vi "TemperatureControl.vi"(8 "error in (no error)":errorcluster, 11 "VISA resource name":refnum<visa-resource-name>="iTC") -> (0 "error out":errorcluster)   [LabVIEW 2021]
uses:
  controls/iTCsetCtrl.ctl
  controls/iTCreadCtrl.ctl
  <vilib>/Instr/_visa.llb/VISA Open Access Mode.ctl
  <vilib>/Utility/file.llb/Write Delimited Spreadsheet (string).vi
panel:
  in  "FilePath":path
  in  "Every (s)":dbl=60.0
  in  "Save Log":bool
  out "Waveform Chart":T1(graph)
  out "Signals":string[](array[string])=["PT1 (K)", "PT2 (K)", "Sample_T (K)", "VTI_T (K)", "Needle Valve (%)", "VTI Heater P", "Sample Heater P ", "VTI Pressure (mBar)"]
  out "Temperature Readings":dbl[](array[numeric])
  in  "Setpoint":dbl
  in  "iTCreadCtrl":T2
  in  "iTCSetCtrl":T3
  in  "Set":bool
  in  "Refresh Time (ms)":i32=100
  in  "Quit":bool
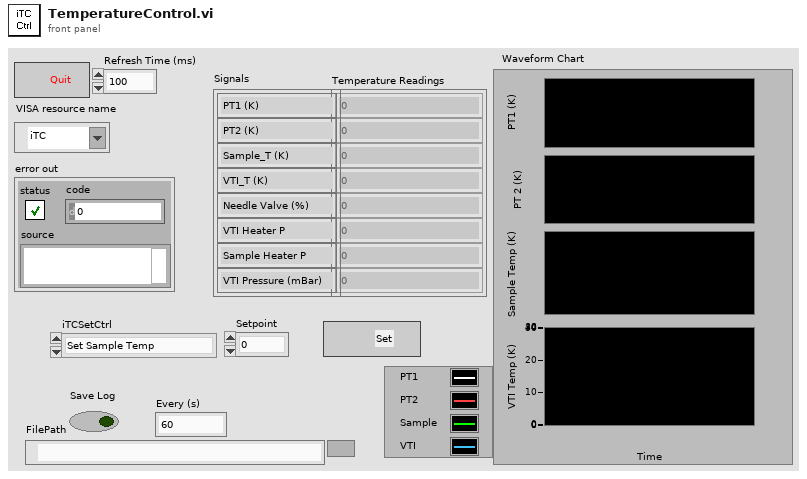
[diagram p1: front panel]
types:
  T1 = cluster{"number":dbl, "number":dbl, "number":dbl, "number":dbl}
  T2 = typedef "iTCreadCtrl.ctl" = enum16{"PT1 Temp", "PT2 Temp", "Sample Temp", "VTI Temp", "Needle Valve", "VTI Heater Power", "Sample Heater Power", "VTI Pressure"}
  T3 = typedef "iTCsetCtrl.ctl" = enum16{"Set Sample Temp", "Set VTI Temp", "Set Needle Valve", "Set VTI Heater Power", "Set Sample Heater Power", "Set VTI Pressure"}
  T4 = typedef "VISA Open Access Mode.ctl" = u32
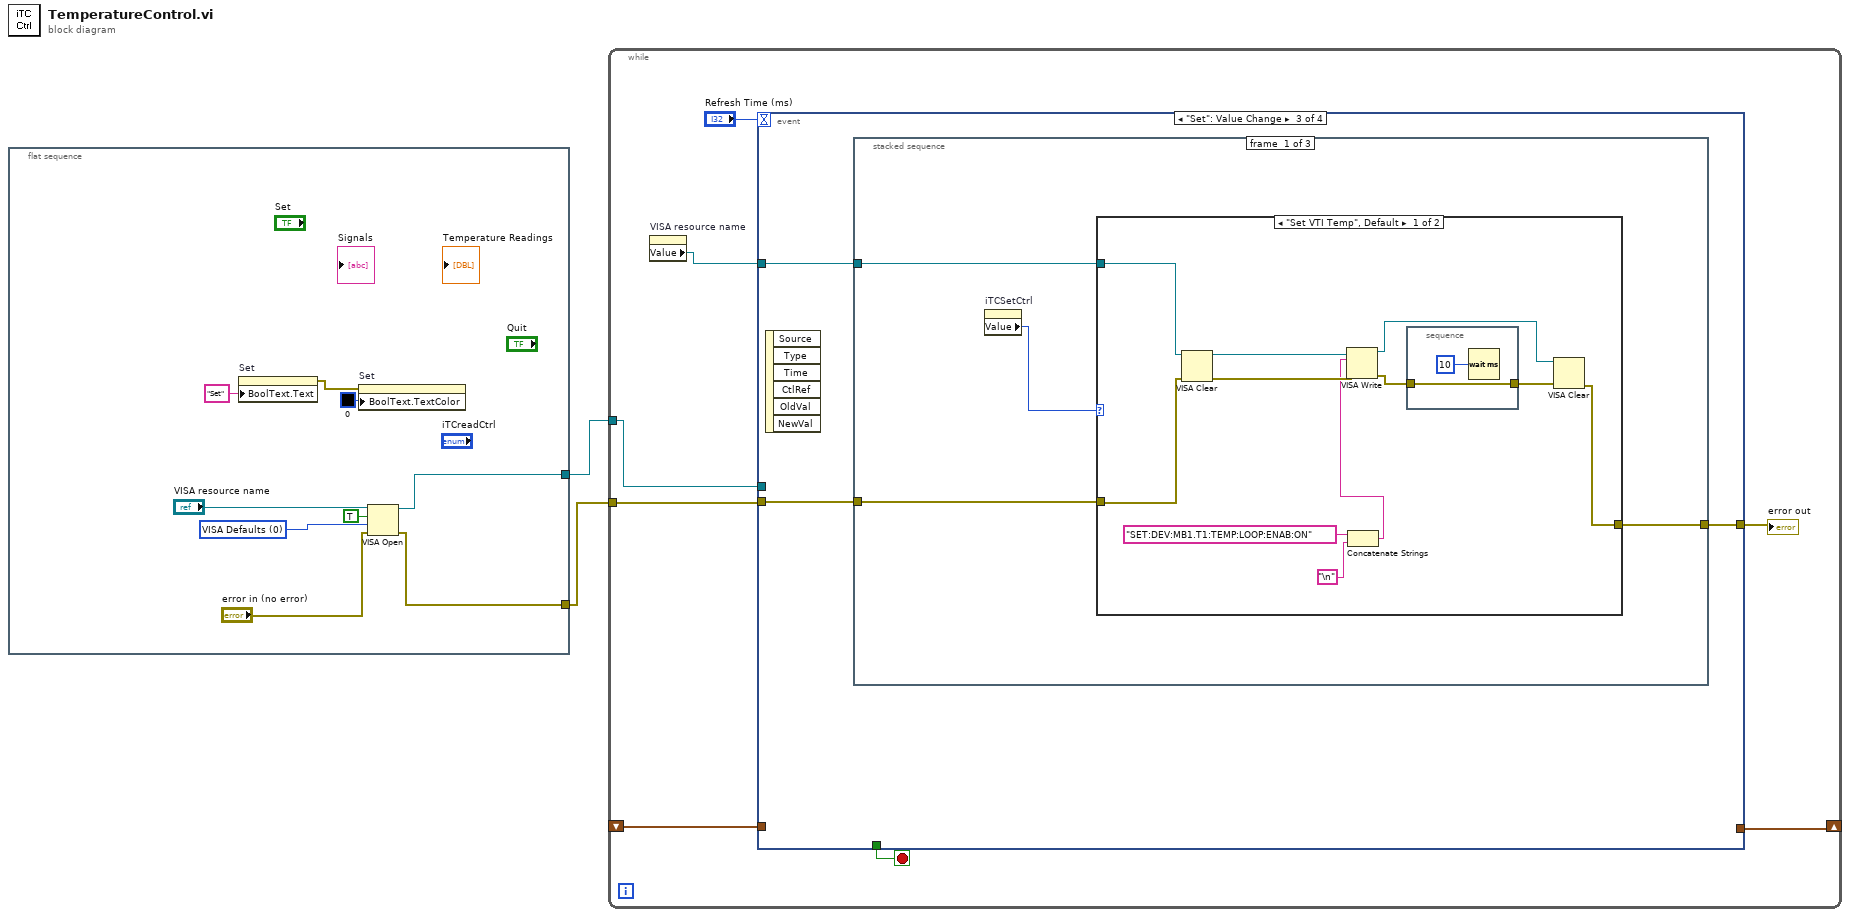
[diagram p0: block diagram]
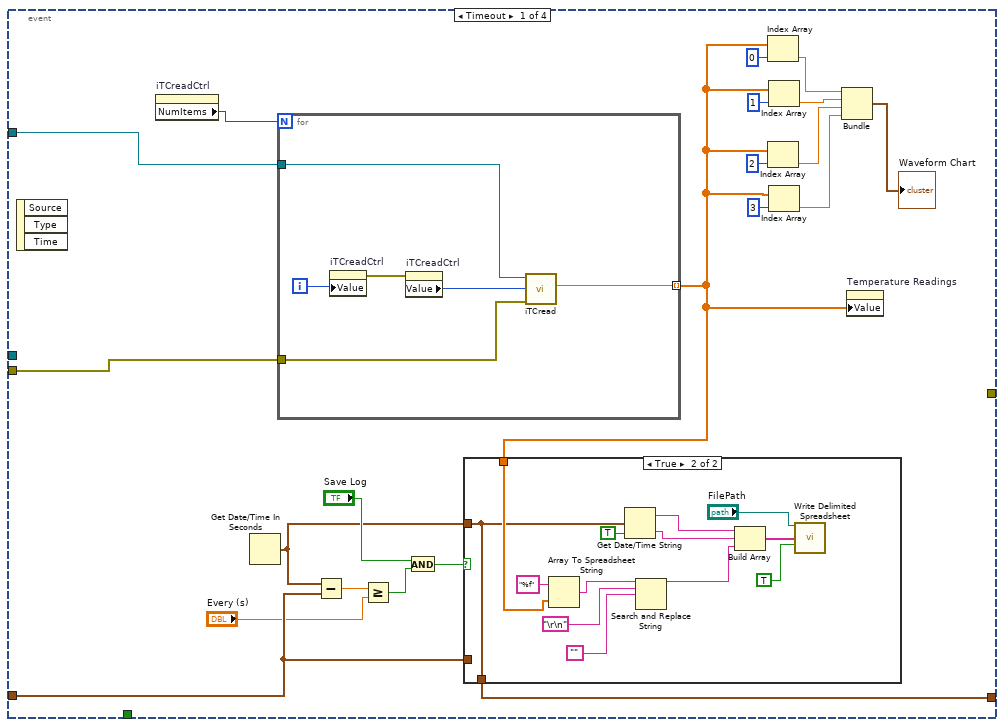
[diagram p2: hidden frame]
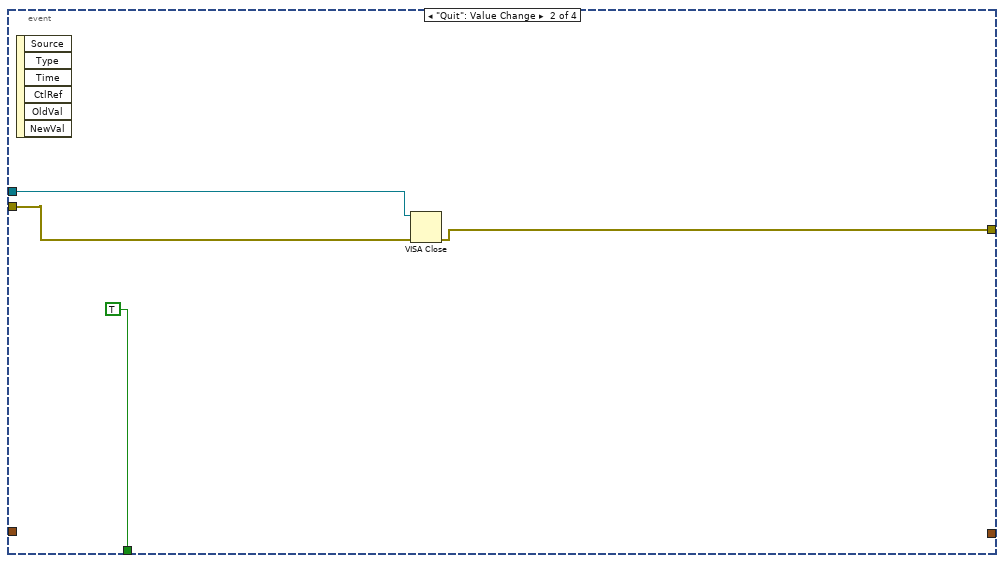
[diagram p4: hidden frame]
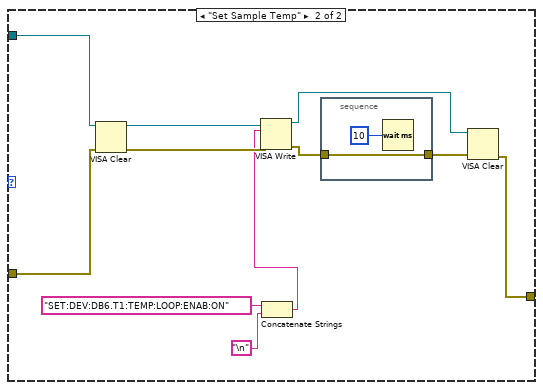
[diagram p5: hidden frame]
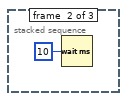
[diagram p6: hidden frame]
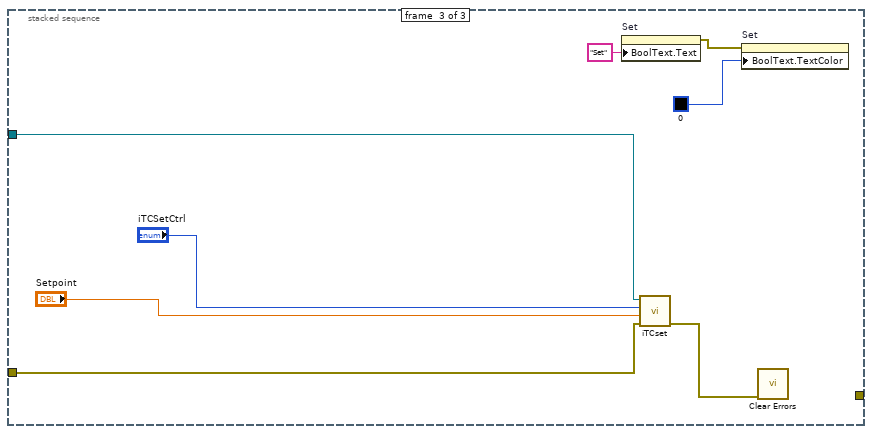
[diagram p7: hidden frame]
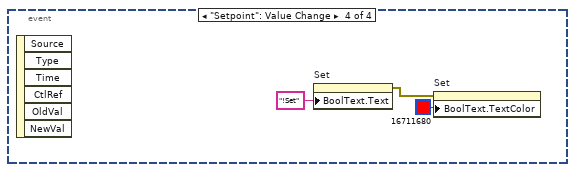
[diagram p8: hidden frame]
diagram:
  n1 = flat-sequence {
    tunnel: [w7] -> w2
    tunnel: [w4] -> w1
    frame #0 {
      w3 = T4 0 items=["VISA Defaults"=0, "Exclusive Lock"=1, "Load Configured Settings"=4] ("Access Mode")
      n2 = property on="Set" class="Bool (strict)"("BoolText.Text"="Set" ("Boolean Text.Text")) -> (error out=w11:errorcluster)  [unwired: 2 in, 1 out]
      n3 = property on="Set" class="Bool (strict)"(error in=w11, "BoolText.TextColor"=u32 0 ("Boolean Text.Colors:BG Color")) -> ()  [unwired: 1 in, 2 out]
      n4 = VISA Open(duplicate session (F)=TRUE, access mode=w3, error in (no error)="error in (no error)", VISA resource name="VISA resource name") -> (VISA resource name=w4:refnum<visa-resource-name>, error out=w7:errorcluster)  [unwired: 1 in]
    }
  }
  n5 = while {
    tunnel: w2 -> [w18]
    tunnel: w1 -> [w15]
    shift-right: [w13] -> _
    shift-left: _ -> [w12]
    stop <- w17 stop-if-true
    n6 = property on="VISA resource name" class="VISAName"() -> ("Value"=w14:refnum<visa-resource-name>)  [unwired: 2 in, 2 out]
    n7 = event shown="[2] \"Set\": Value Change" {
      selector: _ -> [_ _ _ _]
      dyn-events: _ -> [_ _ _ _]
      timeout: "Refresh Time (ms)" -> [_ _ _ _]
      tunnel: w18 -> [w40 w63 w65 _]
      tunnel: [_ w62 w67 _] -> w16
      tunnel: w14 -> [w39 _ w66 _]
      tunnel: [_ TRUE _ _] -> w17
      tunnel: w15 -> [_ w61 _ _]
      tunnel: [w26 _ _ _] -> w13
      tunnel: w12 -> [w25 _ _ _]
      event Timeout {
        n8 = event-data() -> ()  [unwired: 1 in, 3 out]
        n9 = property on="iTCreadCtrl" class="Enum (strict)"() -> ("NumItems"=w38:u32)  [unwired: 2 in, 2 out]
        n10 = Get Date/Time In Seconds() -> (seconds since 1Jan1904=w27:timestamp)
        n11 = for {
          N: w38 -> [_]
          tunnel: w40 -> [w60]
          tunnel: w39 -> [w59]
          tunnel: [w55] -> w20 mode=indexing
          i -> [w58]
          n12 = property on="iTCreadCtrl" class="Enum (strict)"("Value"=w58) -> (error out=w57:errorcluster)  [unwired: 2 in, 1 out]
          n13 = property on="iTCreadCtrl" class="Enum (strict)"(error in=w57) -> ("Value"=w56:T2)  [unwired: 1 in, 2 out]
          n14 = call "iTCread.vi"("VISA resource name"=w59, "iTCreadCtrl"=w56, "error in (no error)"=w60) -> ("number"=w55:dbl)  [unwired: 4 in, 3 out]
        }
        n15 = Subtract(x=w27, y=w25) -> (x-y=w24:dbl)
        n16 = Greater Or Equal?(x=w24, y="Every (s)") -> (x >= y?=w22:bool)
        n17 = And(x="Save Log", y=w22) -> (x .and. y?=w21:bool)
        n18 = case shown="True" w21 {
          tunnel: w27 -> [_ w49]
          tunnel: [w41 w49] -> w26
          tunnel: w25 -> [w41 _]
          tunnel: w20 -> [_ w54]
          frame False {
          }
          frame True {
            n19 = Array To Spreadsheet String(array=w54, 3:"%f" ("format string")) -> (spreadsheet string=w52:string)  [unwired: 1 in]
            n20 = Get Date/Time String(seconds (now)=w49, want seconds? (F)=TRUE ("UTC format")) -> (date string=w47:string, time string=w46:string)  [unwired: 1 in]
            n21 = Search and Replace String(input string=w52, search string="\r\n", replace string="" ("replace string (\"\")")) -> (result string=w45:string)  [unwired: 5 in, 3 out]
            n22 = Build Array(w47, w46, w45) -> (w43:string[])
            n23 = call-poly <vilib>:"Write Delimited Spreadsheet.vi"("file path (dialog if empty)"="FilePath", "1D data"=w43, "append to file? (new file:F)"=TRUE) -> ()  [unwired: 11 in, 2 out]
          }
        }
        n24 = Index Array(array=w20, index=0) -> (element=w33:dbl)
        n25 = Index Array(array=w20, index=2) -> (element=w31:dbl)
        n26 = Index Array(array=w20, index=1) -> (element=w32:dbl)
        n27 = Index Array(array=w20, index=3) -> (element=w30:dbl)
        n28 = Bundle("number"=w33, "number"=w32, "number"=w31, "number"=w30) -> (→"Waveform Chart":T1)  [unwired: 1 in]
        n29 = property on="Temperature Readings" class="Arr (strict)"("Value"=w20) -> ()  [unwired: 2 in, 2 out]
      }
      event "Quit": Value Change {
        n30 = event-data() -> ()  [unwired: 1 in, 6 out]
        n31 = VISA Close(VISA resource name=w61, error in (no error)=w63) -> (error out=w62:errorcluster)
      }
      event "Set": Value Change {
        n32 = event-data() -> ()  [unwired: 1 in, 6 out]
        n33 = stacked-sequence {
          tunnel: [w68 _ _] -> w67
          tunnel: w66 -> [w70 _ w106]
          tunnel: w65 -> [w69 _ w105]
          frame #0 {
            n34 = property on="iTCSetCtrl" class="Enum (strict)"() -> ("Value"=w71:T3)  [unwired: 2 in, 2 out]
            n35 = case shown="\"Set VTI Temp\", Default" w71 {
              tunnel: w70 -> [w73 w95]
              tunnel: w69 -> [w74 w94]
              tunnel: [w72 w91] -> w68
              frame "Set VTI Temp", Default {
                n36 = VISA Clear(VISA resource name=w73, error in (no error)=w74) -> (VISA resource name out=w82:refnum<visa-resource-name>, error out=w81:errorcluster)
                n37 = Concatenate Strings("SET:DEV:MB1.T1:TEMP:LOOP:ENAB:ON" ("string"), "\n") -> (w80:string)
                n38 = VISA Write(VISA resource name=w82, write buffer=w80, error in (no error)=w81) -> (VISA resource name out=w77:refnum<visa-resource-name>, error out=w79:errorcluster)  [unwired: 1 out]
                n39 = stacked-sequence {
                  tunnel: w79 -> [w84]
                  tunnel: [w84] -> w78
                  frame #0 {
                    n40 = Wait (ms)(milliseconds to wait=u32 10) -> ()  [unwired: 1 out]
                  }
                }
                n41 = VISA Clear(VISA resource name=w77, error in (no error)=w78) -> (error out=w72:errorcluster)  [unwired: 1 out]
              }
              frame "Set Sample Temp" {
                n42 = VISA Clear(VISA resource name=w95, error in (no error)=w94) -> (VISA resource name out=w93:refnum<visa-resource-name>, error out=w92:errorcluster)
                n43 = Concatenate Strings("SET:DEV:DB6.T1:TEMP:LOOP:ENAB:ON" ("string"), "\n") -> (w88:string)
                n44 = VISA Write(VISA resource name=w93, write buffer=w88, error in (no error)=w92) -> (VISA resource name out=w85:refnum<visa-resource-name>, error out=w87:errorcluster)  [unwired: 1 out]
                n45 = stacked-sequence {
                  tunnel: w87 -> [w97]
                  tunnel: [w97] -> w86
                  frame #0 {
                    n46 = Wait (ms)(milliseconds to wait=u32 10) -> ()  [unwired: 1 out]
                  }
                }
                n47 = VISA Clear(VISA resource name=w85, error in (no error)=w86) -> (error out=w91:errorcluster)  [unwired: 1 out]
              }
            }
          }
          frame #1 {
            n48 = Wait (ms)(milliseconds to wait=u32 10) -> ()  [unwired: 1 out]
          }
          frame #2 {
            n49 = property on="Set" class="Bool (strict)"("BoolText.Text"="Set" ("Boolean Text.Text")) -> (error out=w101:errorcluster)  [unwired: 2 in, 1 out]
            n50 = call "iTCset.vi"("error in (no error)"=w105, "Set Point"="Setpoint", "iTCSetCtrl"="iTCSetCtrl", "VISA resource name"=w106) -> ("error out"=w104:errorcluster)  [unwired: 4 in, 3 out]
            n51 = property on="Set" class="Bool (strict)"(error in=w101, "BoolText.TextColor"=u32 0 ("Boolean Text.Colors:BG Color")) -> ()  [unwired: 1 in, 2 out]
            n52 = call <vilib>:"Clear Errors.vi"("error in (no error)"=w104) -> ()  [unwired: 5 in, 2 out]
          }
        }
      }
      event "Setpoint": Value Change {
        n53 = event-data() -> ()  [unwired: 1 in, 6 out]
        n54 = property on="Set" class="Bool (strict)"("BoolText.Text"="!Set" ("Boolean Text.Text")) -> (error out=w108:errorcluster)  [unwired: 2 in, 1 out]
        n55 = property on="Set" class="Bool (strict)"(error in=w108, "BoolText.TextColor"=u32 16711680 ("Boolean Text.Colors:BG Color")) -> ()  [unwired: 1 in, 2 out]
      }
    }
    "error out" <- w16
  }
